vi "Write.vi"(8 "error in (no error)":errorcluster, 10 "element":variant, 11 "NetworkStreamWriter in":refnum<class "NetworkStreamWriter.lvclass">) -> (0 "error out":errorcluster, 3 "NetworkStreamWriter out":refnum<class "NetworkStreamWriter.lvclass">)   [LabVIEW 2012, in "NetworkStreamWriter.lvclass"]
doc: "Writes the requested value to an internal queue, which will be sent across the network asynchronously by the WriterDaemon.\n\nJared Kirschner, 2012."
uses:
  NetworkStreamWriter.lvclass
  Shared/TimeStampedMessage.ctl
  NetworkStreamWriter.lvclass/NetworkStreamWriter.ctl
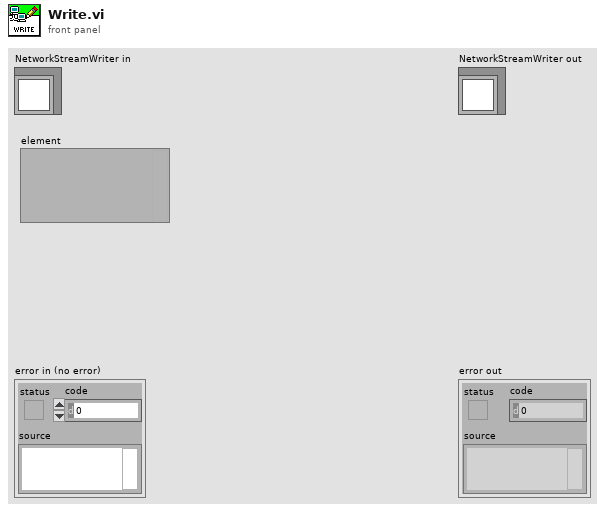
[diagram p1: front panel]
types:
  T1 = typedef "TimeStampedMessage.ctl" = cluster{"Data":variant, "Time Stamp":timestamp}
  T2 = typedef "TimeStampedMessageQueue.ctl" = refnum<queue>
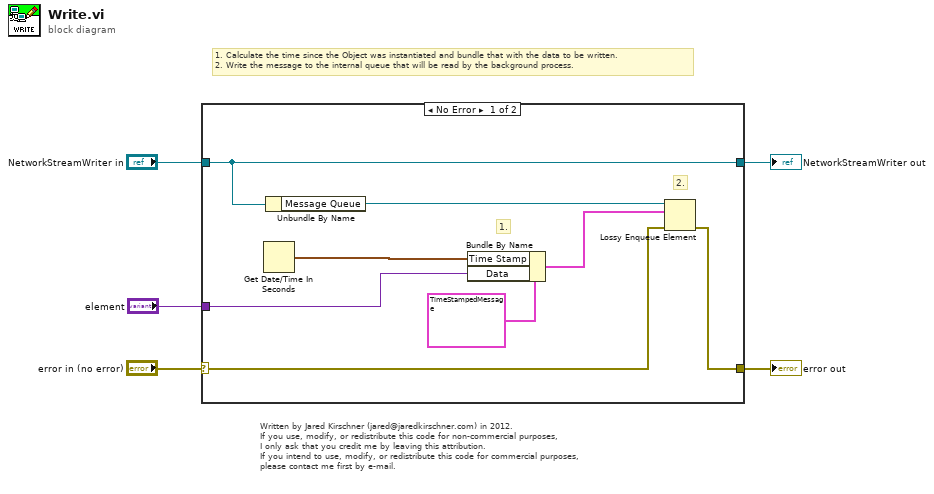
[diagram p0: block diagram]
diagram:
  # "1. Calculate the time since the Object was instantiated and bundle that with the data to be written.\n2. Write the message to the internal queue that will be read by the background process."
  # "Written by Jared Kirschner (jared@jaredkirschner.com) in 2012.\nIf you use, modify, or redistribute this code for non-commercial purposes,\nI only ask that you credit me by leaving this attribution.\nIf you intend to use, modify, or redistribute this code for commercial purposes,\nplease contact me first by e-mail."
  n1 = case shown="No Error" "error in (no error)" {
    selector: "error in (no error)" -> [w9 w14]
    tunnel: [w10 w14] -> w5
    tunnel: [w13 w15] -> w4
    tunnel: "NetworkStreamWriter in" -> [w13 w15]
    tunnel: "element" -> [w8 _]
    frame No Error {
      # "2."
      # "1."
      n2 = Get Date/Time In Seconds() -> (seconds since 1Jan1904=w7:timestamp)
      n3 = Unbundle By Name(w13) -> ("Message Queue"=w12:T2)
      n4 = Bundle By Name(cluster=T1 {"Data"=variant, "Time Stamp"=timestamp(0 s since 1904-01-01)} ("Message"), "Time Stamp"=w7, "Data"=w8) -> (w11:T1)
      n5 = Lossy Enqueue Element(queue=w12, element=w11, error in (no error)=w9) -> (error out=w10:errorcluster)  [unwired: 3 out]
    }
    frame Error {
    }
  }
  "error out" <- w5
  "NetworkStreamWriter out" <- w4
